vi "Get Environment Variable.vi"(8 "error in (no error)":errorcluster, 11 "Environment Variable Name":string) -> (0 "error out":errorcluster, 3 "Variable Value":string)   [LabVIEW 2019]
uses:
  <vilib>/Utility/error.llb/whitespace.ctl
  <vilib>/ErrorRing/Error Ring.xnode
  <vilib>/Utility/error.llb/Error Cluster From Error Code.vi
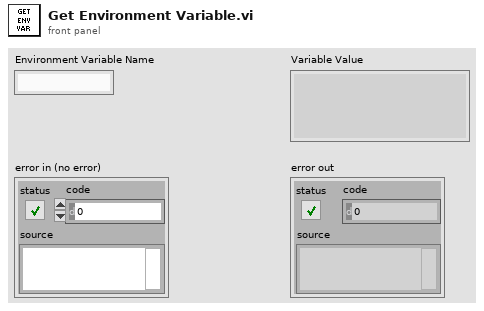
[diagram p1: front panel]
types:
  T1 = typedef "whitespace.ctl" = u16
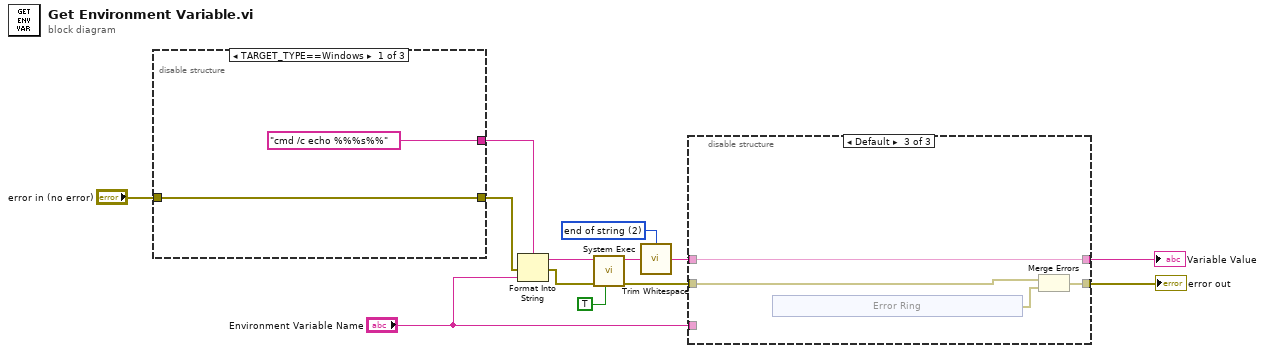
[diagram p0: block diagram]
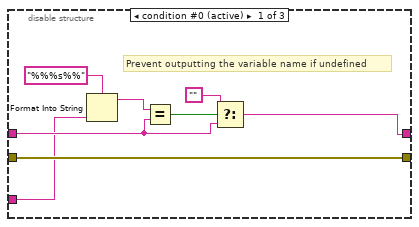
[diagram p2: hidden frame]
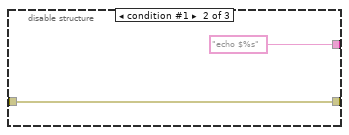
[diagram p4: hidden frame]
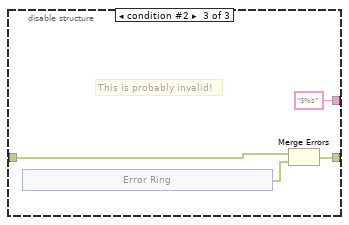
[diagram p5: hidden frame]
diagram:
  w1 = T1 2 items=["both", "start of string", "end of string"] ("location (both)")
  n1 = disable-structure shown="TARGET_TYPE==Windows" {
    disable-tunnel: ["cmd /c echo %%%s%%" "echo $%s" "$%s"] -> w4
    disable-tunnel: [w14 w16 w19] -> w10
    disable-tunnel: "error in (no error)" -> [w14 w16 w20]
    frame condition #0 (active) {
    }
    frame condition #1 {
    }
    frame condition #2 {
      # "This is probably invalid!"
      n2 = xnode "Error Ring"() -> ("error out"=w18:errorcluster)
      n3 = Merge Errors(w20, w18) -> (w19:errorcluster)
    }
  }
  n4 = Format Into String(format string=w4, error in=w10, "Environment Variable Name") -> (resulting string=w13:string, error out=w11:errorcluster)  [unwired: 1 in]
  n5 = call <vilib>:"System Exec.vi"("run minimized? (F)"=TRUE, "error in (no error)"=w11, "command line"=w13) -> ("error out"=w8:errorcluster, "standard output"=w6:string)  [unwired: 5 in, 2 out]
  n6 = call <vilib>:"Trim Whitespace.vi"("string"=w6, "location (both)"=w1) -> ("trimmed string"=w2:string)
  n7 = disable-structure shown="Default" {
    disable-tunnel: [w33 w35 w38] -> w7
    disable-tunnel: w8 -> [w33 w35 w39]
    disable-tunnel: w2 -> [w31 w34 w36]
    disable-tunnel: [w29 w34 w36] -> w5
    disable-tunnel: "Environment Variable Name" -> [w28 _ _]
    frame condition #0 (active) {
      # "Prevent outputting the variable name if undefined"
      n8 = Format Into String(format string="%%%s%%", w28) -> (resulting string=w26:string)  [unwired: 2 in, 1 out]
      n9 = Equal?(x=w26, y=w31) -> (x = y?=w32:bool)
      n10 = Select(t="", s=w32, f=w31) -> (s? t:f=w29:string)
    }
    frame condition #1 {
      # "Think this is fine?"
    }
    frame condition #2 {
      n11 = xnode "Error Ring"() -> ("error out"=w37:errorcluster)
      n12 = Merge Errors(w39, w37) -> (w38:errorcluster)
    }
  }
  "Variable Value" <- w5
  "error out" <- w7
